vi "Apply_RF.vi"(0 "I- index":dbl, 4 "I+ index":dbl, 5 "RF Proportional to intensity":bool, 6 "RF Target Position":i32, 7 "RF indicator":bool, 8 "RF Power":dbl, 9 "rho0":dbl[](array[numeric]), 10 "rho-":dbl[](array[numeric]), 11 "rho+":dbl[](array[numeric])) -> (1 "rho- out":dbl[](array[numeric]), 2 "rho0 out":dbl[](array[numeric]), 3 "rho+ out":dbl[](array[numeric]))   [LabVIEW 2018]
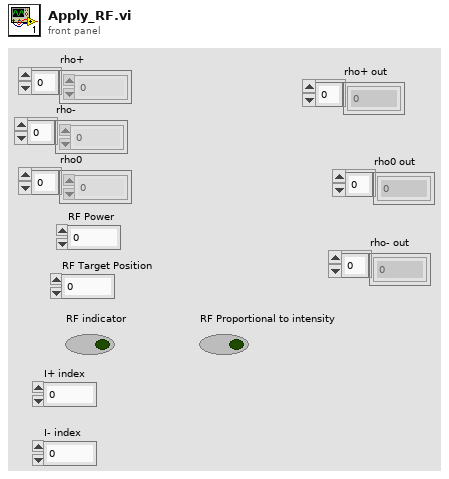
[diagram p1: front panel]
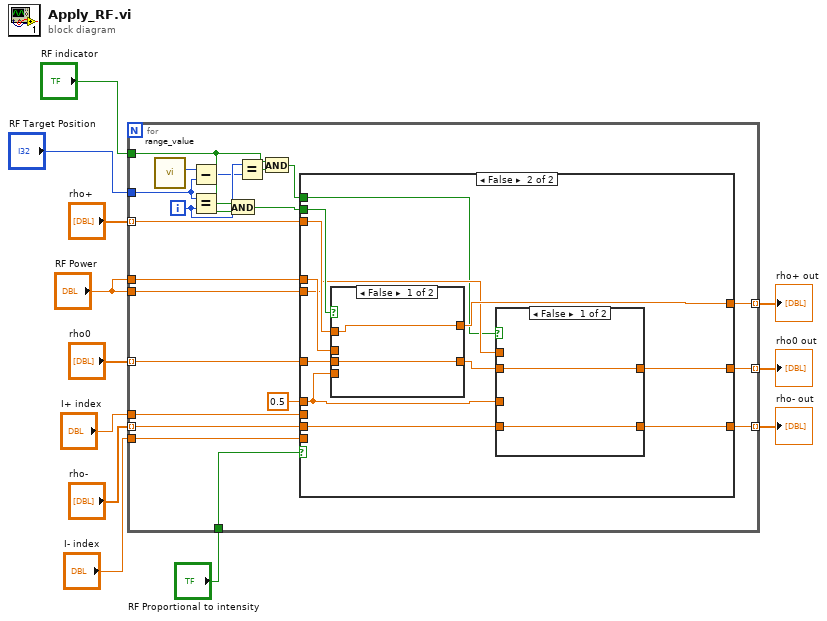
[diagram p0: block diagram]
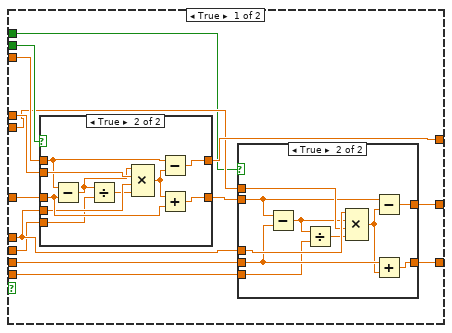
[diagram p2: hidden frame]
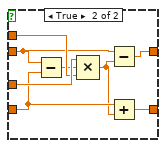
[diagram p5: hidden frame]
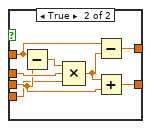
[diagram p6: hidden frame]
diagram:
  n1 = for {
    tunnel: "rho+" -> [w33] mode=indexing
    tunnel: "rho0" -> [w25] mode=indexing
    tunnel: "rho-" -> [w26] mode=indexing
    tunnel: "RF Power" -> [w30]
    tunnel: "RF Target Position" -> [w21]
    tunnel: [w31] -> w8 mode=indexing
    tunnel: [w23] -> w7 mode=indexing
    tunnel: [w28] -> w6 mode=indexing
    tunnel: "RF indicator" -> [w18]
    tunnel: "RF Power" -> [w27]
    tunnel: "I+ index" -> [w16]
    tunnel: "I- index" -> [w15]
    tunnel: "RF Proportional to intensity" -> [w14]
    i -> [w20]
    n2 = call "range_value.vi"() -> ("NumBins"=w22:i32)  [unwired: 10 in, 1 out]
    n3 = Subtract(x=w22, y=w21) -> (x-y=w13:i32)
    n4 = Equal?(x=w21, y=w20) -> (x = y?=w32:bool)
    n5 = And(x=w32, y=w18) -> (x .and. y?=w29:bool)
    n6 = Equal?(x=w20, y=w13) -> (x = y?=w19:bool)
    n7 = And(x=w18, y=w19) -> (x .and. y?=w17:bool)
    n8 = case shown="False" w14 {
      tunnel: w33 -> [w47 w83]
      tunnel: [w46 w82] -> w31
      tunnel: w30 -> [w45 w81]
      tunnel: w29 -> [w44 w80]
      tunnel: [w43 w79] -> w28
      tunnel: w27 -> [w42 w78]
      tunnel: w26 -> [w41 w77]
      tunnel: w25 -> [w40 w76]
      tunnel: 0.5 -> [w39 w75]
      tunnel: [w37 w73] -> w23
      tunnel: w17 -> [w36 w72]
      tunnel: w16 -> [w35 _]
      tunnel: w15 -> [w34 _]
      frame True {
        n9 = case shown="True" w44 {
          tunnel: w47 -> [w61 w69]
          tunnel: w40 -> [w60 w66]
          tunnel: [w61 w68] -> w46
          tunnel: [w60 w67] -> w38
          tunnel: w45 -> [_ w71]
          tunnel: w39 -> [_ w65]
          tunnel: w35 -> [_ w63]
          frame False {
          }
          frame True {
            n10 = Subtract(x=w69, y=w66) -> (x-y=w62:dbl)
            n11 = Divide(x=w62, y=w63) -> (x/y=w64:dbl)
            n12 = Compound Arithmetic op=MULTIPLY(w62, w71, w65, w64) -> (w70:dbl)
            n13 = Subtract(x=w69, y=w70) -> (x-y=w68:dbl)
            n14 = Add(x=w70, y=w66) -> (x+y=w67:dbl)
          }
        }
        n15 = case shown="True" w36 {
          tunnel: [w48 w59] -> w43
          tunnel: w39 -> [_ w58]
          tunnel: w42 -> [_ w57]
          tunnel: w41 -> [w48 w56]
          tunnel: w38 -> [w49 w54]
          tunnel: [w49 w53] -> w37
          tunnel: w34 -> [_ w50]
          frame False {
          }
          frame True {
            n16 = Subtract(x=w54, y=w56) -> (x-y=w51:dbl)
            n17 = Divide(x=w51, y=w50) -> (x/y=w52:dbl)
            n18 = Compound Arithmetic op=MULTIPLY(w58, w51, w57, w52) -> (w55:dbl)
            n19 = Subtract(x=w54, y=w55) -> (x-y=w53:dbl)
            n20 = Add(x=w56, y=w55) -> (x+y=w59:dbl)
          }
        }
      }
      frame False {
        n21 = case shown="False" w80 {
          tunnel: w83 -> [w95 w100]
          tunnel: w76 -> [w94 w97]
          tunnel: [w95 w99] -> w82
          tunnel: [w94 w98] -> w74
          tunnel: w81 -> [_ w102]
          tunnel: w75 -> [_ w96]
          frame False {
          }
          frame True {
            n22 = Subtract(x=w100, y=w97) -> (x-y=w103:dbl)
            n23 = Compound Arithmetic op=MULTIPLY(w103, w102, w96) -> (w101:dbl)
            n24 = Subtract(x=w100, y=w101) -> (x-y=w99:dbl)
            n25 = Add(x=w101, y=w97) -> (x+y=w98:dbl)
          }
        }
        n26 = case shown="False" w72 {
          tunnel: [w84 w93] -> w79
          tunnel: w75 -> [_ w92]
          tunnel: w78 -> [_ w91]
          tunnel: w77 -> [w84 w89]
          tunnel: w74 -> [w85 w87]
          tunnel: [w85 w86] -> w73
          frame False {
          }
          frame True {
            n27 = Subtract(x=w87, y=w89) -> (x-y=w90:dbl)
            n28 = Compound Arithmetic op=MULTIPLY(w92, w90, w91) -> (w88:dbl)
            n29 = Subtract(x=w87, y=w88) -> (x-y=w86:dbl)
            n30 = Add(x=w89, y=w88) -> (x+y=w93:dbl)
          }
        }
      }
    }
  }
  "rho+ out" <- w8
  "rho0 out" <- w7
  "rho- out" <- w6
